vi "dvp Vi Set Record Param.vi"(10 "quality":u32, 11 "recordName":string) -> (2 "function return":u32(ring), 3 "recordName out":string)   [LabVIEW 2018, in "LabViewDVPCamera.lvlib"]
doc: "LabviewDvp2Api dvpStatus dvpViSetRecordParam(char *recordName,dvpUint32 quality=100);"
uses:
  LabViewDVPCamera.lvlib
  LabViewDVPCamera/LabViewDVPCamera.dll
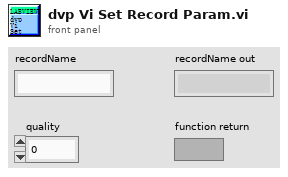
[diagram p1: front panel]
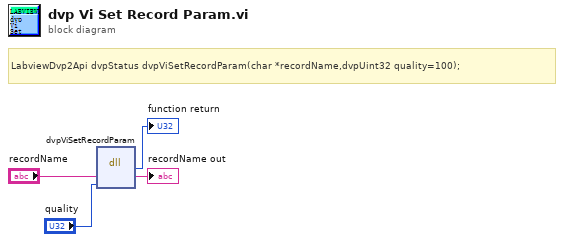
[diagram p0: block diagram]
diagram:
  # "LabviewDvp2Api dvpStatus dvpViSetRecordParam(char *recordName,dvpUint32 quality=100);"
  n1 = dll-call lib="C:/Program Files (x86)/DVP2 Labview cn 64/Sample/LabViewDVPCamera/LabViewDVPCamera.*" fn="dvpViSetRecordParam"("recordName"="recordName", "quality"="quality") -> (→"function return":u32, "recordName"=→"recordName out":string)  [unwired: 4 in, 2 out]
